vi "Configure Reading Hold.vi"(7 "Enable Hold (F: Disable)":bool, 8 "error in (no error)":errorcluster, 9 "Hold Count (5)":i32=5, 10 "Hold Window (1%)":dbl=1.0, 11 "VISA resource name":refnum<visa-resource-name>) -> (0 "error out":errorcluster, 3 "VISA resource name out":refnum<visa-resource-name>)   [LabVIEW 2016, in "Keithley 2182.lvlib"]
doc: "Configures the 2182's Reading Hold (autosettle) feature. Reading Hold is used to screen out readings that are not within a specified reading window.\n\nWith hold enabled (HOLD annunciator on), the first processed reading becomes the \"seed\" reading and operation loops back within the device action block. After the next reading is processed, it is checked to see if it is within the selected hold window of the \"seed\" reading. If the reading is within the window, operation again loops back within the device action block. This looping continues until the specified number (2 to 100) of consecutive readings are within the window. If one of the readings is not within the window, the instrument acquires a new \"seed\" reading and the hold process continues.\n\n<B>Note:</B>\nHold can only be used with Channel 1. Whenever Hold is enabled, Channel 2 becomes inoperative."
uses:
  Keithley 2182.lvlib
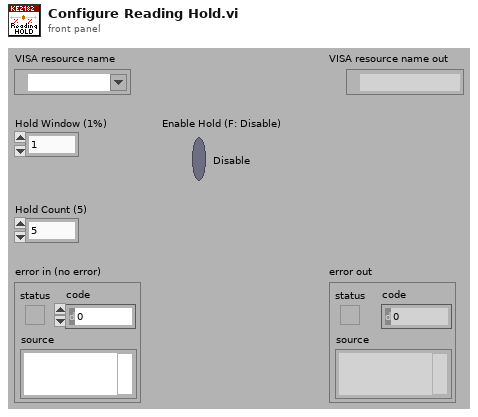
[diagram p1: front panel]
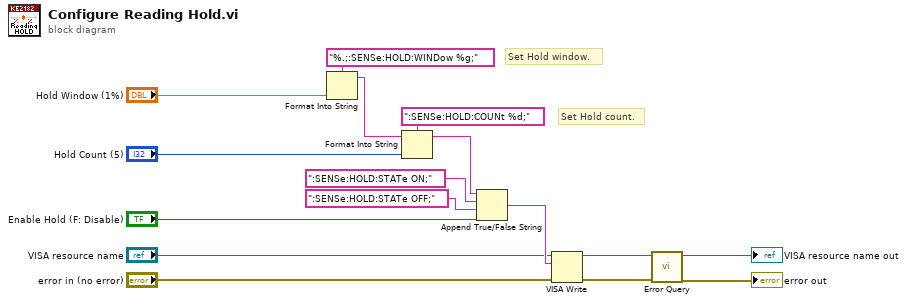
[diagram p0: block diagram]
diagram:
  # "Set Hold count."
  # "Set Hold window."
  n1 = Format Into String(format string="%.;:SENSe:HOLD:WINDow %g;", "Hold Window (1%)") -> (resulting string=w14:string)  [unwired: 2 in, 1 out]
  n2 = Format Into String(format string=":SENSe:HOLD:COUNt %d;", initial string=w14, "Hold Count (5)") -> (resulting string=w11:string)  [unwired: 1 in, 1 out]
  n3 = Append True/False String(1:"Enable Hold (F: Disable)", 2:":SENSe:HOLD:STATe OFF;", 3:":SENSe:HOLD:STATe ON;", 4:w11) -> (0:w7:string)
  n4 = VISA Write(VISA resource name="VISA resource name", write buffer=w7, error in (no error)="error in (no error)") -> (VISA resource name out=w4:refnum<visa-resource-name>, error out=w3:errorcluster)  [unwired: 1 out]
  n5 = call "Error Query.vi"("error in (no error)"=w3, "VISA resource name"=w4) -> ("error out"=→"error out":errorcluster, "VISA resource name out"=→"VISA resource name out":refnum<visa-resource-name>)  [unwired: 6 in, 2 out]
